vi "pct.vi"() -> ()   [LabVIEW 2016]
panel:
  out "Pict Ring":u16(ring)
  in  "Boolean 3":bool
  in  "Numeric":dbl
  out "Tab Control":enum32{"Page 1", "Page 2", "Page 3"}(tab)
  out "Gauge":dbl(knob) scale=0.0..10.0
  in  "Thermometer":dbl(slide) scale=0.0..100.0
  in  "Boolean":bool
  out "Boolean 2":bool
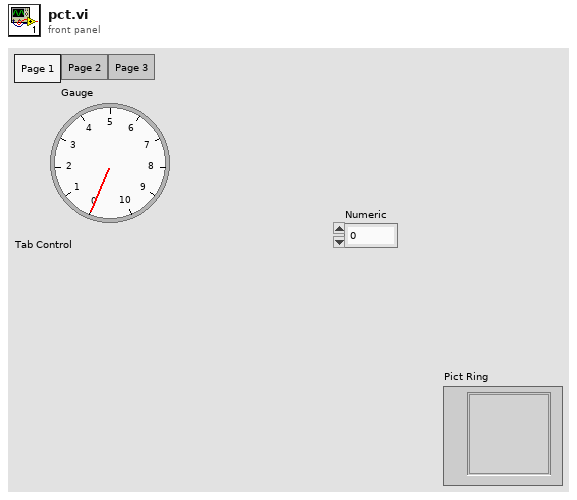
[diagram p1: front panel]
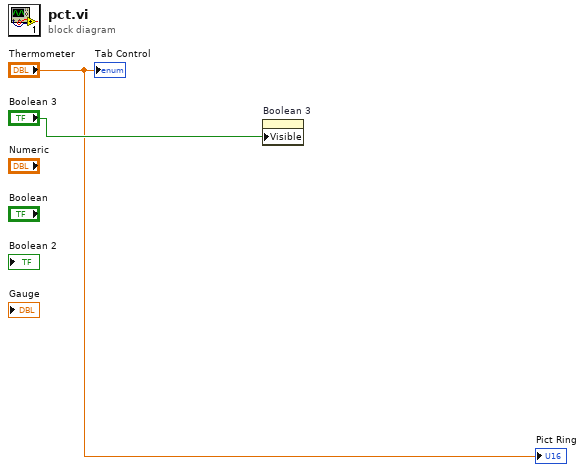
[diagram p0: block diagram]
diagram:
  n1 = property on="Boolean 3" class="Bool (strict)"("Visible"="Boolean 3") -> ()  [unwired: 2 in, 2 out]
  "Tab Control" <- "Thermometer"
  "Pict Ring" <- "Thermometer"
